vi "Flip_Flop.vi"(8 "E1":bool, 11 "E0":bool) -> (3 "A0":bool)   [LabVIEW 2020]
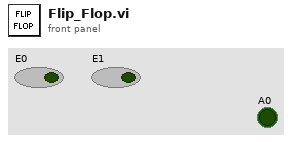
[diagram p1: front panel]
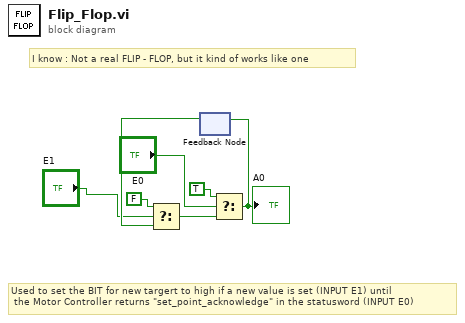
[diagram p0: block diagram]
diagram:
  # "Used to set the BIT for new targert to high if a new value is set (INPUT E1) until\n the Motor Controller returns \"set_point_acknowledge\" in the statusword (INPUT E0)"
  # "I know : Not a real FLIP - FLOP, but it kind of works like one"
  n1 = feedback #1() -> (w6:bool)  [unwired: 1 in]
  n2 = Select(t=FALSE, s="E1", f=w6) -> (s? t:f=w5:bool)
  n3 = Select(t=TRUE, s="E0", f=w5) -> (s? t:f=w3:bool)
  "A0" <- w3
  n4 = feedback-in #1(w3) -> ()
